vi "intial single psu test.vi"() -> ()   [LabVIEW 2020]
panel:
  in  "?":bool
  out "Current Voltage":dbl
  in  "ANODE VOLTAGE":dbl(slide) min=0.0 max=3000.0 step=0.183 scale=3.0..3000.0 scale format="%#_7f"
  in  "Anode Enable":bool
  out "NI 9263":dbl
  in  "Ki":dbl
  in  "Kd":dbl
  in  "Kp":dbl
  # "at Anode"
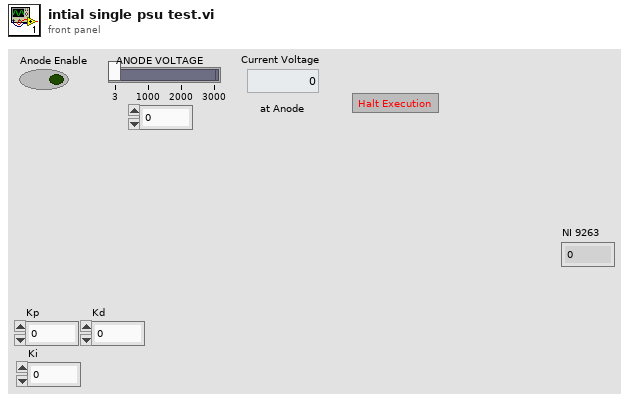
[diagram p1: front panel]
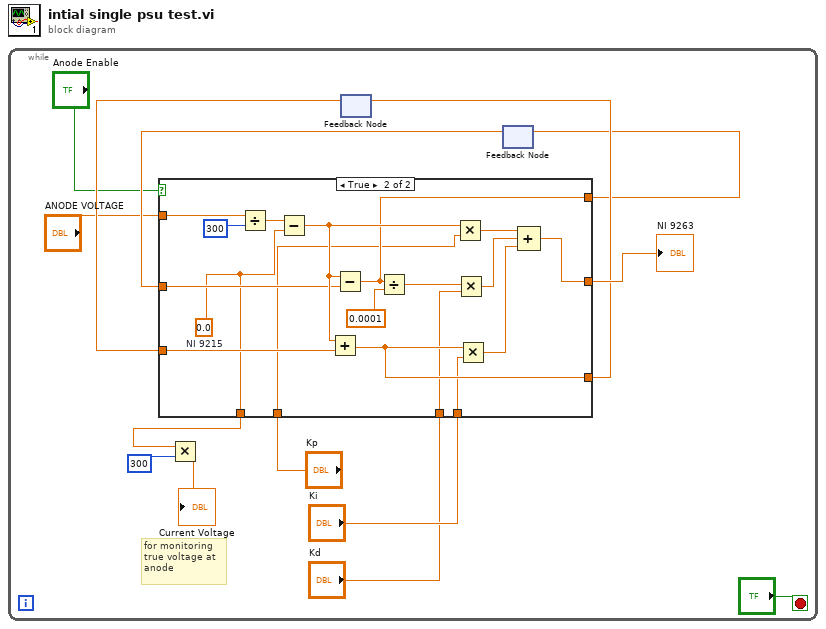
[diagram p0: block diagram]
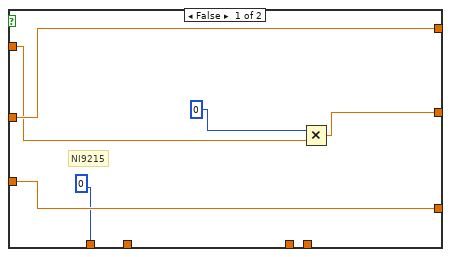
[diagram p2: hidden frame]
diagram:
  n1 = while {
    stop <- "?" stop-if-true
    # "for monitoring \ntrue voltage at\nanode"
    n2 = feedback #1() -> (w13:dbl)  [unwired: 1 in]
    n3 = feedback #2() -> (w14:dbl)  [unwired: 1 in]
    n4 = case shown="True" "Anode Enable" {
      tunnel: w14 -> [w20 w30]
      tunnel: [w20 w29] -> w3
      tunnel: w13 -> [w19 w28]
      tunnel: [w19 w27] -> w8
      tunnel: "ANODE VOLTAGE" -> [w17 w26]
      tunnel: [w16 w25] -> w11
      tunnel: "Kp" -> [_ w24]
      tunnel: "Ki" -> [_ w23]
      tunnel: "Kd" -> [_ w22]
      tunnel: [0 w21] -> w4
      frame False {
        # "NI9215"
        n5 = Multiply(x=0, y=w17) -> (x*y=w16:dbl)
      }
      frame True {
        w21 = 0.0  # NI 9215
        n6 = Divide(x=w26, y=300) -> (x/y=w32:dbl)
        n7 = Subtract(x=w32, y=w21) -> (x-y=w37:dbl)
        n8 = Add(x=w37, y=w28) -> (x+y=w27:dbl)
        n9 = Subtract(x=w37, y=w30) -> (x-y=w29:dbl)
        n10 = Divide(x=w29, y=0.0001) -> (x/y=w34:dbl)
        n11 = Multiply(x=w37, y=w24) -> (x*y=w35:dbl)
        n12 = Multiply(x=w34, y=w22) -> (x*y=w31:dbl)
        n13 = Multiply(x=w27, y=w23) -> (x*y=w36:dbl)
        n14 = Compound Arithmetic op=ADD(w35, w31, w36) -> (w25:dbl)
      }
    }
    "NI 9263" <- w11
    n15 = Multiply(x=w4, y=300) -> (x*y=→"Current Voltage":dbl)
    n16 = feedback-in #1(w8) -> ()
    n17 = feedback-in #2(w3) -> ()
  }
